vi "Error Dialog.vi"(8 "error in":errorcluster, 10 "Data":variant, 11 "QDMH in":refnum<class "QDMH.lvclass">) -> (0 "error out":errorcluster, 2 "Halt?":bool, 3 "QDMH out":refnum<class "QDMH.lvclass">)   [LabVIEW 2023, in "QDMH.lvlib" / "QDMH.lvclass"]
uses:
  QDMH.lvclass
  Custom Controls/QDMH Message.ctl
panel:
  in  "Halt":bool
  in  "Abort":bool
  out "Alert:":string
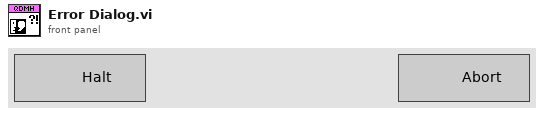
[diagram p1: front panel]
types:
  T1 = typedef "QDMH.lvlib/QDMH.lvclass/QDMH Message.ctl" = cluster{"State":string, "Data":variant}
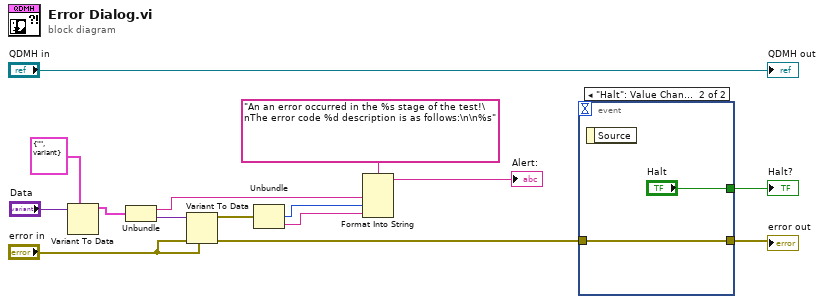
[diagram p0: block diagram]
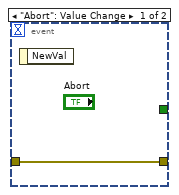
[diagram p2: hidden frame]
diagram:
  n1 = Variant To Data(type=T1 {"State"="", "Data"=variant} ("Message"), Variant="Data") -> (data=w13:T1)  [unwired: 1 in, 1 out]
  n2 = Unbundle(w13) -> ("State"=w10:string, "Data"=w12:variant)
  n3 = Variant To Data(error in="error in", type="error in", Variant=w12) -> (data=w9:errorcluster, error out=w3:errorcluster)
  n4 = Unbundle(w9) -> ("code"=w8:i32, "source"=w7:string)  [unwired: 1 out]
  n5 = Format Into String(format string="An an error occurred in the %s stage of the test!\nThe error code %d description is as follows:\n\n%s", w10, w8, w7) -> (resulting string=→"Alert:":string)  [unwired: 2 in, 1 out]
  n6 = event shown="[1] \"Halt\": Value Change" {
    selector: _ -> [_ _]
    dyn-events: _ -> [_ _]
    timeout: _ -> [_ _]
    tunnel: [_ "Halt"] -> w4
    tunnel: w3 -> [w16 w17]
    tunnel: [w16 w17] -> w2
    event "Abort": Value Change {
      n7 = event-data() -> ()  [unwired: 1 in, 1 out]
    }
    event "Halt": Value Change {
      n8 = event-data() -> ()  [unwired: 1 in, 1 out]
    }
  }
  "error out" <- w2
  "Halt?" <- w4
  "QDMH out" <- "QDMH in"
